vi "Finish.vi"   [LabVIEW 2020]
doc: "This VI is called just before exiting. It is expected to close I/O refnum, save collected data, etc."
uses:
  Globals/Calibration_And_Constant_Globals.vi
  <vilib>/Rock Robotics/WPI/Utilities/WPI_GetSetVariantRefNum.vi
types:
  T1 = typedef "WPI_JoystickDevRef.ctl" = cluster{"Device":T2}
  T2 = typedef "WPI_JoystickDeviceEnum.ctl" = enum16{"USB 0", "USB 1", "USB 2", "USB 3", "USB 4", "USB 5"}
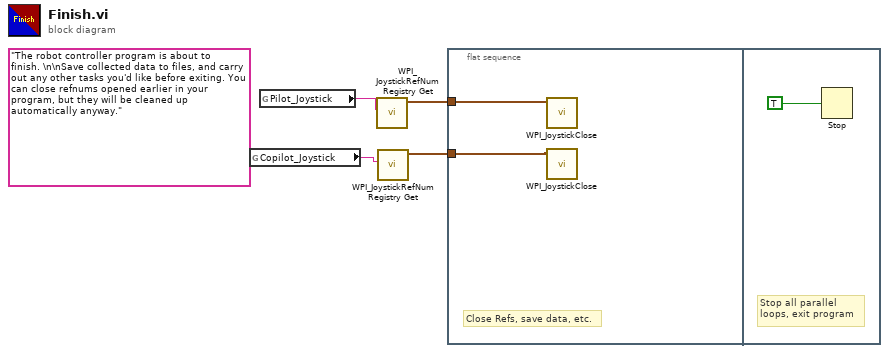
[diagram p0: block diagram]
diagram:
  (unwired) "The robot controller program is about to finish. \n\nSave collected data to files, and carry out any other tasks you'd like before exiting. You can close refnums opened earlier in your program, but they will be cleaned up automatically anyway."
  n1 = global read "Calibration_And_Constant_Globals.vi" "Copilot_Joystick"() -> (w1:string)
  n2 = global read "Calibration_And_Constant_Globals.vi" "Pilot_Joystick"() -> (w3:string)
  n3 = call <vilib>:"WPI_JoystickRefNum Registry Get.vi"("refnum name"=w3) -> ("JoystickDevRef"=w4:T1)  [unwired: 1 in, 9 out]
  n4 = call <vilib>:"WPI_JoystickRefNum Registry Get.vi"("refnum name"=w1) -> ("JoystickDevRef"=w2:T1)  [unwired: 1 in, 9 out]
  n5 = flat-sequence {
    tunnel: w4 -> [w6]
    tunnel: w2 -> [w5]
    frame #0 {
      # "Close Refs, save data, etc."
      n6 = call <vilib>:"WPI_JoystickClose.vi"("JoystickDevRef"=w6) -> ()  [unwired: 11 out]
      n7 = call <vilib>:"WPI_JoystickClose.vi"("JoystickDevRef"=w5) -> ()  [unwired: 11 out]
    }
    frame #1 {
      # "Stop all parallel\nloops, exit program"
      n8 = Stop(stop? (T)=TRUE ("Quit")) -> ()
    }
  }
